vi "PLC.vi"(8 "error in":errorcluster, 10 "Message Queues":T3, 11 "Notifiers":T4) -> (0 "error out":errorcluster)   [LabVIEW 2015, in "PLC.lvlib"]
uses:
  PLC.lvlib
  support/Notifiers/Notifiers.ctl
  support/Message Queue/All Message Queues.ctl
  support/Message Queue/Message Cluster.ctl
  Type definitions/PLC Data.ctl
  DAQ/TypeDefs/DAQ data.ctl
  support/Global names.vi
  <vilib>/Utility/error.llb/Error Cluster From Error Code.vi
  <vilib>/ErrorRing/Error Ring.xnode
  support/Message Queue/Message Queue.lvlib
  Model/Model.lvlib
  DAQ/DAQ.lvlib
  support/Notifiers/Notifiers.lvlib
panel:
  in  "PLC Data":T1={"DAQ data"={"Power switch (DI)"={"Channel"="myDAQ1/port0/line0", "Data"=FALSE}, "Dispose barrel (DI)"={"Channel"="myDAQ1/port0/line1", "Data"=FALSE}, "Pump status (DO)"={"Channel"="myDAQ1/port0/line2", "Data"=FALSE}, "Barrel position (AI)"={"Channel"="myDAQ1/ai0", "Data"=0.0}}, "Run process"=FALSE}
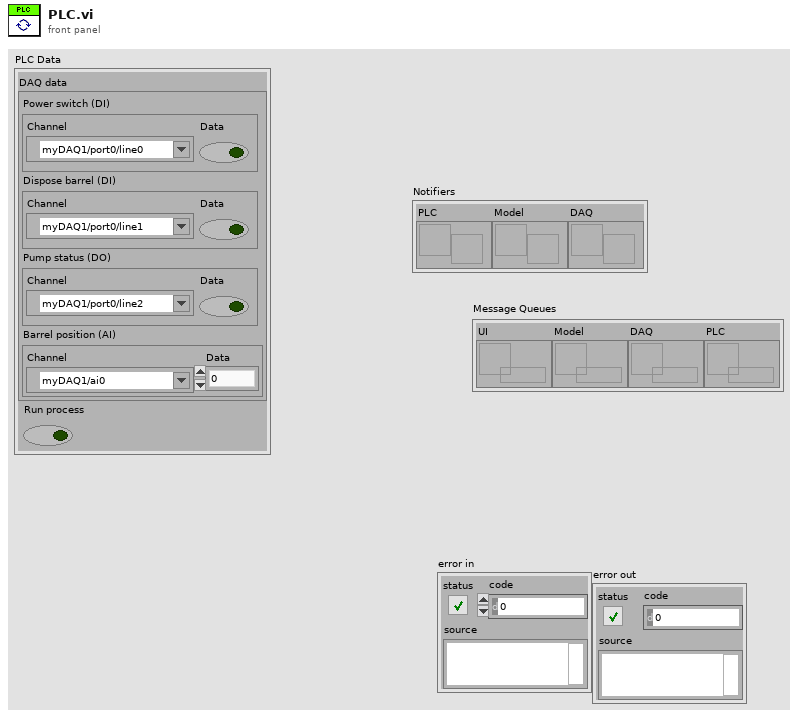
[diagram p1: front panel]
types:
  T1 = typedef "PLC.lvlib/PLC Data.ctl" = cluster{"DAQ data":T2, "Run process":bool}
  T2 = typedef "DAQ.lvlib/DAQ data.ctl" = cluster{"Power switch (DI)":cluster{"Channel":tag, "Data":bool}, "Dispose barrel (DI)":cluster{"Channel":tag, "Data":bool}, "Pump status (DO)":cluster{"Channel":tag, "Data":bool}, "Barrel position (AI)":cluster{"Channel":tag, "Data":dbl}}
  T3 = typedef "Message Queue.lvlib/All Message Queues.ctl" = cluster{"UI":refnum<queue>, "Model":refnum<queue>, "DAQ":refnum<queue>, "PLC":refnum<queue>}
  T4 = typedef "Notifiers.lvlib/Notifiers.ctl" = cluster{"PLC":refnum<notifier>, "Model":refnum<notifier>, "DAQ":refnum<notifier>}
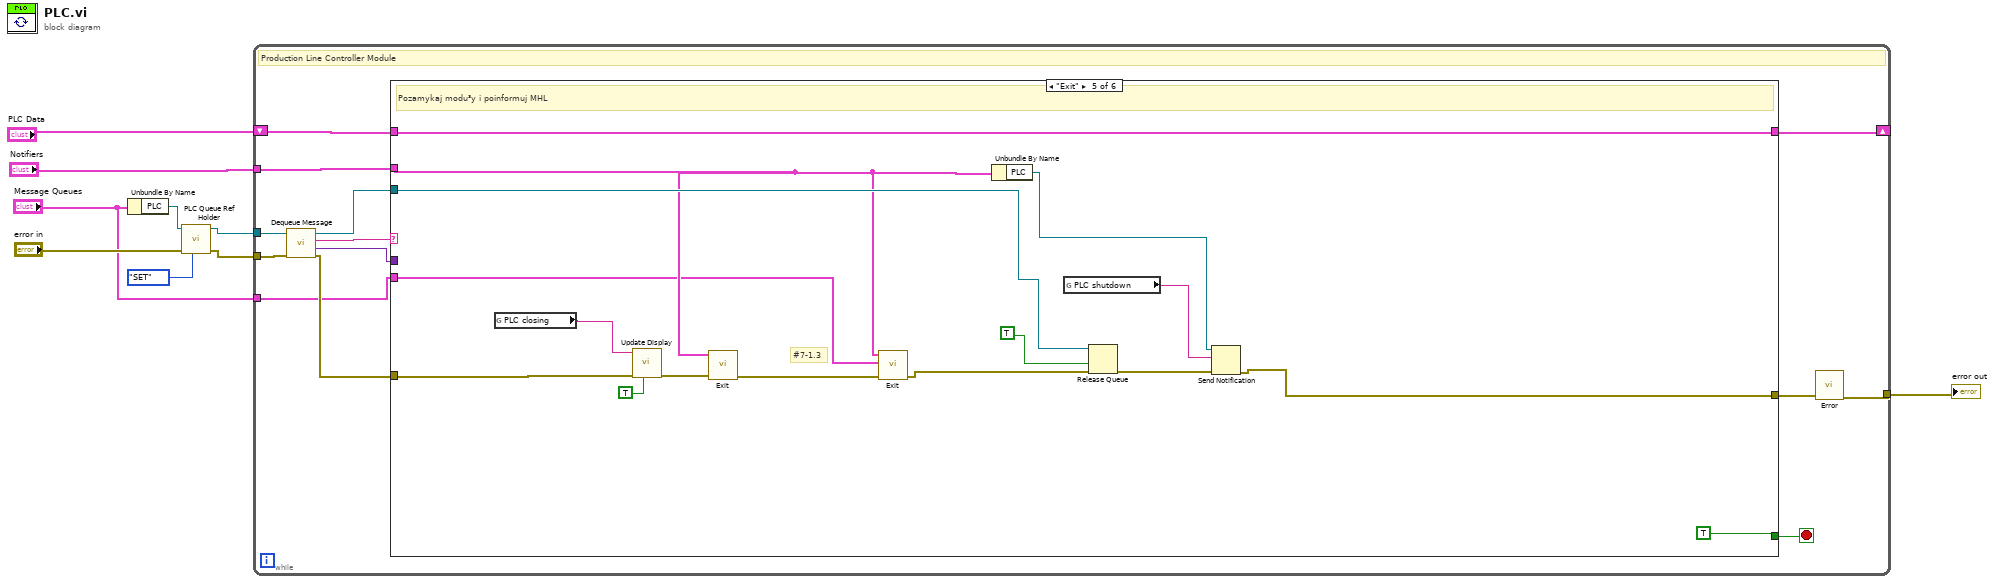
[diagram p0: block diagram]
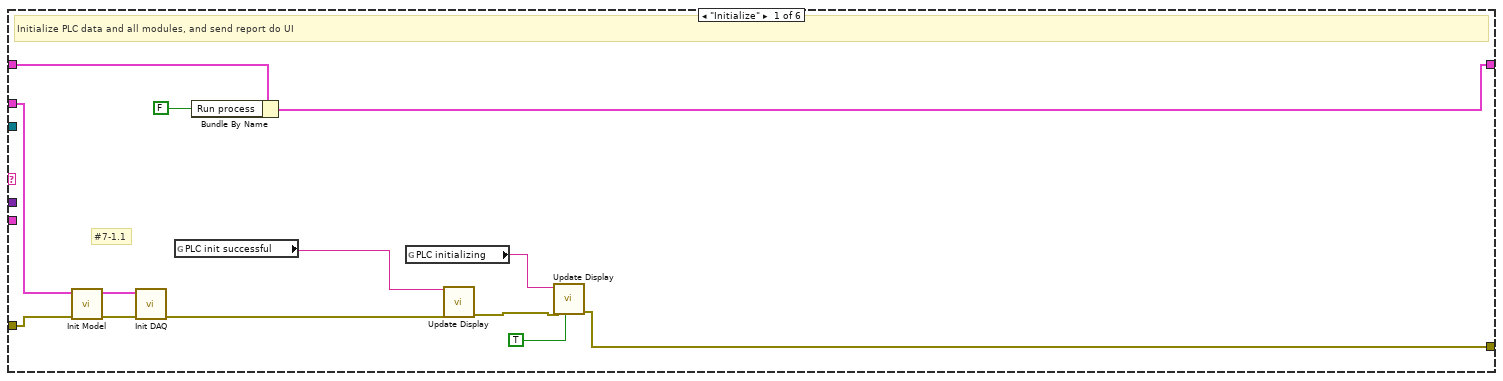
[diagram p2: hidden frame]
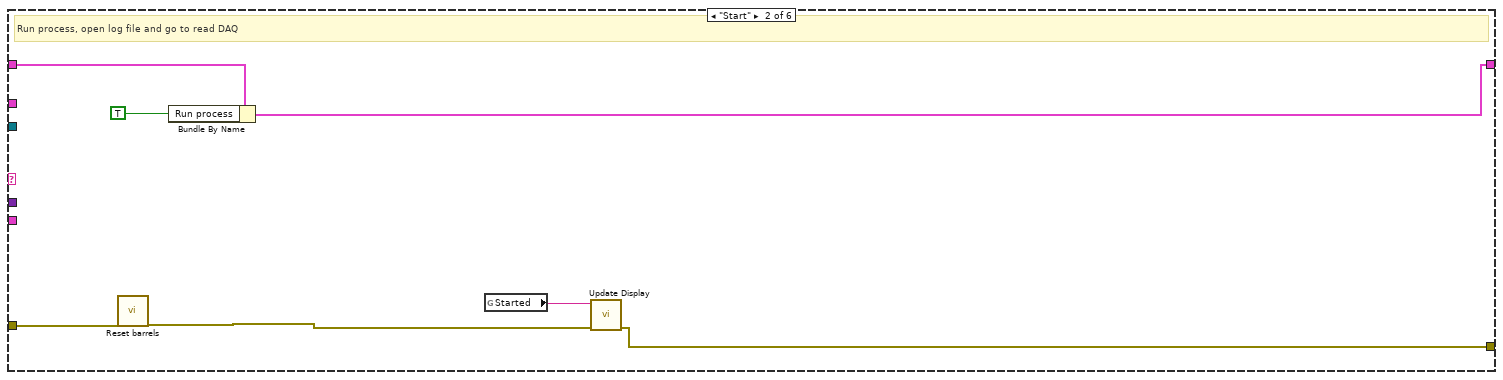
[diagram p3: hidden frame]
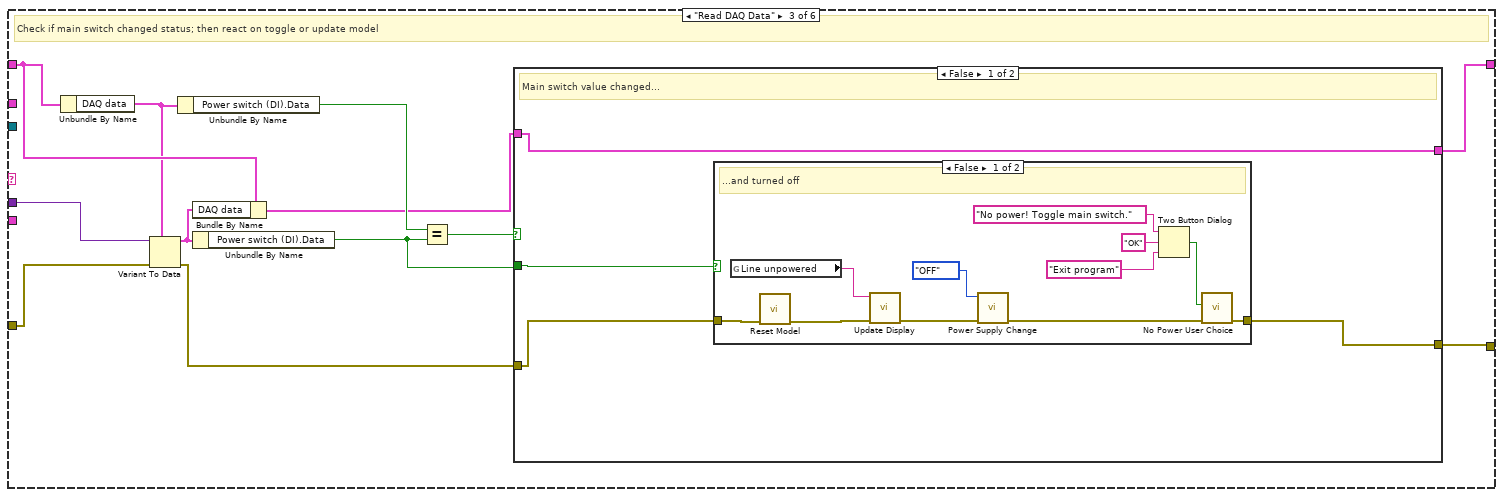
[diagram p4: hidden frame]
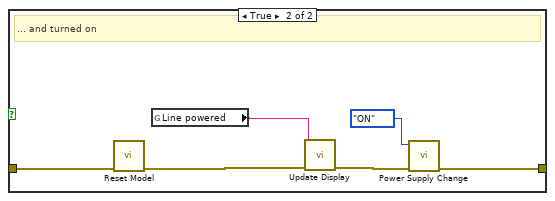
[diagram p5: hidden frame]
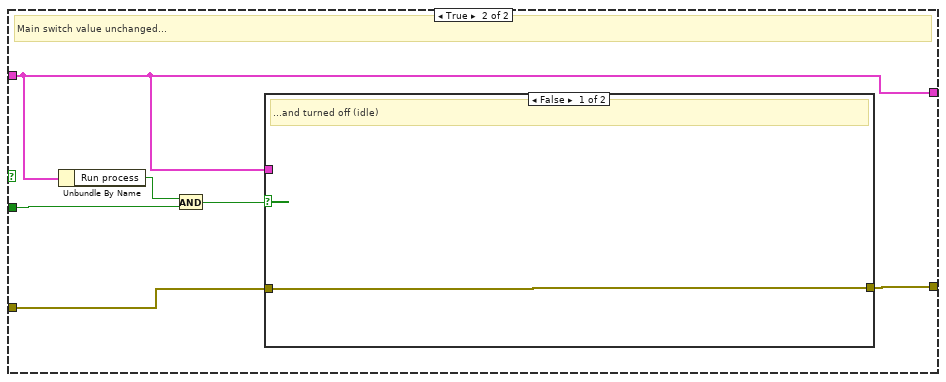
[diagram p6: hidden frame]
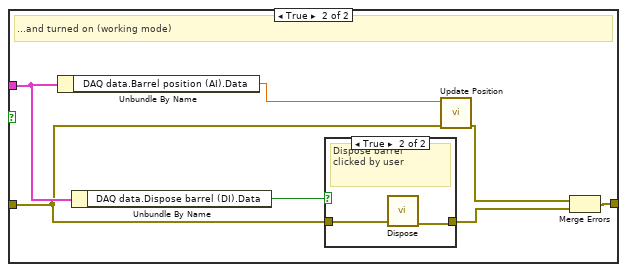
[diagram p7: hidden frame]
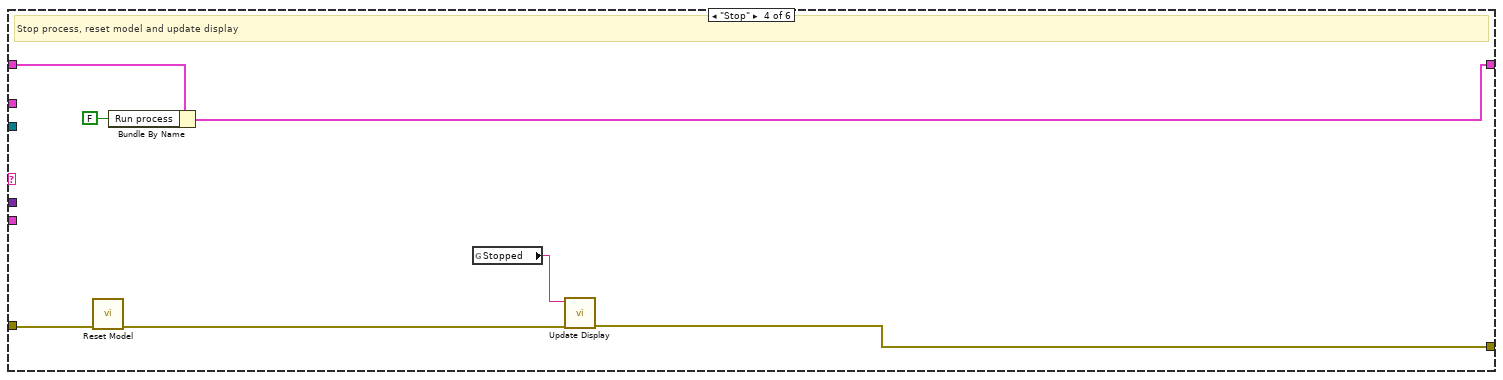
[diagram p9: hidden frame]
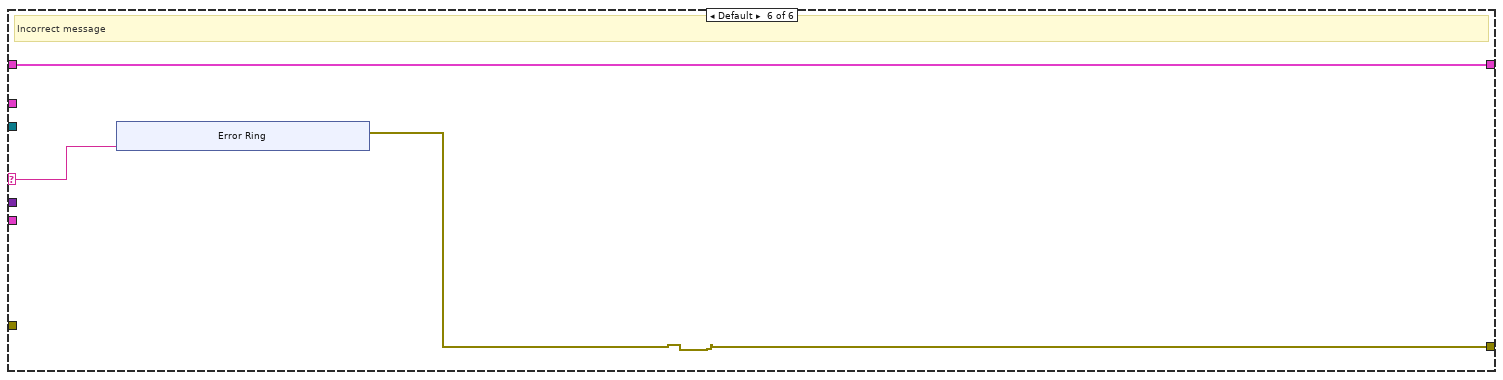
[diagram p10: hidden frame]
diagram:
  n1 = Unbundle By Name("Message Queues") -> ("PLC"=w4:refnum<queue>)
  n2 = call "PLC Queue Ref Holder.vi"("Action"=enum16{"GET", "SET"}."SET", "error in"="error in", "Message Queue In"=w4) -> ("error out"=w5:errorcluster, "Input Message Queue"=w3:refnum<queue>)  [unwired: 7 in]
  n3 = while {
    tunnel: "Notifiers" -> [w22]
    tunnel: w3 -> [w21]
    tunnel: w5 -> [w20]
    tunnel: [w11] -> w9
    tunnel: "Message Queues" -> [w17]
    shift-right: [w15] -> _
    shift-left: "PLC Data" -> [w14]
    stop <- w18 stop-if-true
    # "Production Line Controller Module"
    n4 = call "Dequeue Message.vi"("error in (no error)"=w20, "Message Queue"=w21) -> ("error out"=w19:errorcluster, "Message Data"=w16:variant, "Message"=w10:string, "dup Message Queue"=w13:refnum<queue>)  [unwired: 6 in]
    n5 = case shown="\"Exit\"" w10 {
      selector: w10 -> [_ _ _ _ _ w117]
      tunnel: w22 -> [w33 _ _ _ w101 _]
      tunnel: w19 -> [w32 w37 w53 w95 w104 _]
      tunnel: w13 -> [_ _ _ _ w106 _]
      tunnel: [_ _ _ _ TRUE _] -> w18
      tunnel: [w29 w39 w43 w94 w108 w116] -> w12
      tunnel: w17 -> [_ _ _ _ w100 _]
      tunnel: w16 -> [_ _ w54 _ _ _]
      tunnel: w14 -> [w35 w42 w52 w99 w105 w118]
      tunnel: [w34 w41 w44 w97 w105 w118] -> w15
      frame "Initialize" {
        # "#7-1.1"
        # "Initialize PLC data and all modules, and send report do UI"
        n6 = call "Init Model.vi"("error in"=w32, "Notifiers in"=w33) -> ("error out"=w24:errorcluster, "Notifiers out"=w25:T4)  [unwired: 8 in]
        n7 = call "Init DAQ.vi"("error in"=w24, "Notifiers in"=w25) -> ("error out"=w23:errorcluster)  [unwired: 8 in, 1 out]
        n8 = global read "Global names.vi" "PLC init successful"() -> (w27:string)
        n9 = Bundle By Name(cluster=w35, "Run process"=FALSE) -> (w34:T1)
        n10 = global read "Global names.vi" "PLC initializing"() -> (w26:string)
        n11 = call "Update Display.vi"("error in"=w23, "Message string"=w27) -> ("error out"=w30:errorcluster)  [unwired: 9 in]
        n12 = call "Update Display.vi"("Priority Message? (F)"=TRUE, "error in"=w30, "Message string"=w26) -> ("error out"=w29:errorcluster)  [unwired: 8 in]
      }
      frame "Start" {
        # "Run process, open log file and go to read DAQ"
        n13 = call "Reset barrels.vi"("error in"=w37) -> ("error out"=w36:errorcluster)  [unwired: 10 in]
        n14 = Bundle By Name(cluster=w42, "Run process"=TRUE) -> (w41:T1)
        n15 = global read "Global names.vi" "Started"() -> (w38:string)
        n16 = call "Update Display.vi"("error in"=w36, "Message string"=w38) -> ("error out"=w39:errorcluster)  [unwired: 9 in]
      }
      frame "Read DAQ Data" {
        # "Check if main switch changed status; then react on toggle or update model"
        n17 = Unbundle By Name(w52) -> ("DAQ data"=w51:T2)
        n18 = Variant To Data(error in=w53, type=w51, Variant=w54) -> (data=w47:T2, error out=w45:errorcluster)
        n19 = Unbundle By Name(w51) -> ("Power switch (DI).Data"=w50:bool)
        n20 = Bundle By Name(cluster=w52, "DAQ data"=w47) -> (w46:T1)
        n21 = Unbundle By Name(w47) -> ("Power switch (DI).Data"=w48:bool)
        n22 = Equal?(x=w50, y=w48) -> (x = y?=w49:bool)
        n23 = case shown="False" w49 {
          tunnel: [w58 w80] -> w43
          tunnel: w48 -> [w57 w77]
          tunnel: w46 -> [w55 w76]
          tunnel: w45 -> [w56 w81]
          tunnel: [w55 w76] -> w44
          frame False {
            # "Main switch value changed..."
            n24 = case shown="False" w57 {
              tunnel: [w61 w71] -> w58
              tunnel: w56 -> [w60 w72]
              frame False {
                # "...and turned off"
                n25 = global read "Global names.vi" "Line unpowered"() -> (w59:string)
                n26 = call "Reset Model.vi"("error in"=w60) -> ("error out"=w63:errorcluster)  [unwired: 10 in]
                n27 = call "Update Display.vi"("error in"=w63, "Message string"=w59) -> ("error out"=w65:errorcluster)  [unwired: 9 in]
                n28 = call "Power Supply Change.vi"("error in"=w65, "Power status"=enum16{"OFF", "ON"}."OFF") -> ("error out"=w62:errorcluster)  [unwired: 9 in]
                n29 = Two Button Dialog(message="No power! Toggle main switch.", 1:"Exit program" ("F button name (\"Cancel\")"), 2:"OK" ("button name (\"OK\")")) -> (T button?=w66:bool)
                n30 = call "No Power User Choice.vi"("error in (no error)"=w62, "T button?"=w66) -> ("error out"=w61:errorcluster)  [unwired: 9 in]
              }
              frame True {
                # "... and turned on"
                n31 = call "Reset Model.vi"("error in"=w72) -> ("error out"=w73:errorcluster)  [unwired: 10 in]
                n32 = global read "Global names.vi" "Line powered"() -> (w70:string)
                n33 = call "Update Display.vi"("error in"=w73, "Message string"=w70) -> ("error out"=w75:errorcluster)  [unwired: 9 in]
                n34 = call "Power Supply Change.vi"("error in"=w75, "Power status"=enum16{"OFF", "ON"}."ON") -> ("error out"=w71:errorcluster)  [unwired: 9 in]
              }
            }
          }
          frame True {
            # "Main switch value unchanged..."
            n35 = Unbundle By Name(w76) -> ("Run process"=w78:bool)
            n36 = And(x=w78, y=w77) -> (x .and. y?=w79:bool)
            n37 = case shown="False" w79 {
              tunnel: w76 -> [_ w88]
              tunnel: w81 -> [w82 w87]
              tunnel: [w82 w86] -> w80
              frame False {
                # "...and turned off (idle)"
              }
              frame True {
                # "...and turned on (working mode)"
                n38 = Unbundle By Name(w88) -> ("DAQ data.Barrel position (AI).Data"=w83:dbl)
                n39 = Unbundle By Name(w88) -> ("DAQ data.Dispose barrel (DI).Data"=w89:bool)
                n40 = case shown="True" w89 {
                  tunnel: w87 -> [w90 w92]
                  tunnel: [w90 w91] -> w84
                  frame False {
                  }
                  frame True {
                    # "Dispose barrel\nclicked by user"
                    n41 = call "Dispose.vi"("error in (no error)"=w92) -> ("error out"=w91:errorcluster)  [unwired: 10 in]
                  }
                }
                n42 = call "Update Position.vi"("error in (no error)"=w87, "Position"=w83) -> ("error out"=w85:errorcluster)  [unwired: 9 in]
                n43 = Merge Errors(w85, w84) -> (w86:errorcluster)
              }
            }
          }
        }
      }
      frame "Stop" {
        # "Stop process, reset model and update display"
        n44 = call "Reset Model.vi"("error in"=w95) -> ("error out"=w93:errorcluster)  [unwired: 10 in]
        n45 = Bundle By Name(cluster=w99, "Run process"=FALSE) -> (w97:T1)
        n46 = global read "Global names.vi" "Stopped"() -> (w96:string)
        n47 = call "Update Display.vi"("error in"=w93, "Message string"=w96) -> ("error out"=w94:errorcluster)  [unwired: 9 in]
      }
      frame "Exit" {
        # "#7-1.3"
        # "Pozamykaj modu³y i poinformuj MHL"
        n48 = global read "Global names.vi" "PLC closing"() -> (w110:string)
        n49 = call "Update Display.vi"("Priority Message? (F)"=TRUE, "error in"=w104, "Message string"=w110) -> ("error out"=w107:errorcluster)  [unwired: 8 in]
        n50 = call "Exit.vi"("error in"=w107, "Notifiers"=w101) -> ("error out"=w103:errorcluster)  [unwired: 9 in]
        n51 = call "Exit.vi"("error in"=w103, "Message Queues"=w100, "Notifiers"=w101) -> ("error out"=w102:errorcluster)  [unwired: 8 in]
        n52 = Unbundle By Name(w101) -> ("PLC"=w112:refnum<notifier>)
        n53 = global read "Global names.vi" "PLC shutdown"() -> (w109:string)
        n54 = Release Queue(queue=w106, force destroy? (F)=TRUE, error in (no error)=w102) -> (error out=w114:errorcluster)  [unwired: 2 out]
        n55 = Send Notification(notification=w109, notifier=w112, error in (no error)=w114) -> (error out=w108:errorcluster)  [unwired: 1 out]
      }
      frame Default {
        # "Incorrect message"
        n56 = xnode "Error Ring"("parameter 0"=w117) -> ("error out"=w116:errorcluster)
      }
    }
    n57 = call "Error.vi"("error in"=w12) -> ("error out"=w11:errorcluster)  [unwired: 10 in]
  }
  "error out" <- w9
